vi "Automatic Frequency Linearization.vi"() -> ()   [LabVIEW 2014]
panel:
  out "1) Falling Max-Min error Graph":cluster{dbl[], dbl[]}(graph)
  out "2) Rising Max-Min error Graph":cluster{dbl[], dbl[]}(graph)
  out "2) Rising Max-Min error %":dbl
  out "1) Falling Max-Min error %":dbl
  in  "Active PolyFit of Mean Freq":bool
  out "Triangular skewtri generated from min factor":dbl[](graph)
  in  "Sample /Modulation Frequency":enum32{"40MHz/32KHz", "30MHz/24Khz"}(radio)=enum."30MHz/24Khz"
  in  "Scaling factor":dbl=1.0
  out "Rising Min Factor":dbl
  out "Falling Min Factor":dbl
  out "Rising Min DevStd%":dbl
  out "Falling Min DevStd%":dbl
  out "Fine?":bool
  out "Ok?":bool
  in  "#MeanMeasuraments":i32=50
  in  "StopValue":dbl=0.2
  in  "stop":bool
  out "Mean  FREQUENCY Curve Falling":dbl[](graph)
  out "Mean FREQUENCY Curve Rising":dbl[](graph)
  out "Current Skew Tri":dbl[](graph)
  out "Current Mul factor":dbl
  out "Current iteration (Countdown)":dbl
  out "Rising<= 1%":bool
  out "Falling<= 1%":bool
  in  "DeltaFactor":dbl=0.01
  in  "Initial Factor Mul":dbl=0.35
  out "2) Rising StdDev % Graph":cluster{dbl[], dbl[]}(graph)
  out "1) Falling StdDev % Graph":cluster{dbl[], dbl[]}(graph)
  out "2) Rising Std Dev %":dbl
  out "1) Falling Std Dev %":dbl
  out "2) Rising Signal (Last)":dbl[](graph)
  out "1) Falling Signal (Last)":dbl[](graph)
  in  "#LinMesuraments":i32=20
  # "OFFLINE SETUP"
  # "CURRENT ITERATION"
  # "Fattore moltiplicativo"
  # "Numero di misure su cui calcolare la curva delle frequenze medie con triangolo dritto"
  # "Numero di misurazioni\n su cui mediare durante la\nlinearizzazione"
  # "Optimal Factor Rising: 0.33    with Falling curve: 0.294"
  # "Optimal Factor Falling: 0.22/0.23"
  # "Fattore moltiplicativo\nIniziale"
  # "Passo del fattore\nmoltiplicativo"
  # "Fattore moltiplicativo\nFinale"
  # "%"
  # "%"
  # "FINAL RESULTS"
  # "Andamento della deviazione standard percentuale in funzione del fattore moltiplicativo"
  # "%"
  # "%"
  # "min 0,27"
  # "min 0,16"
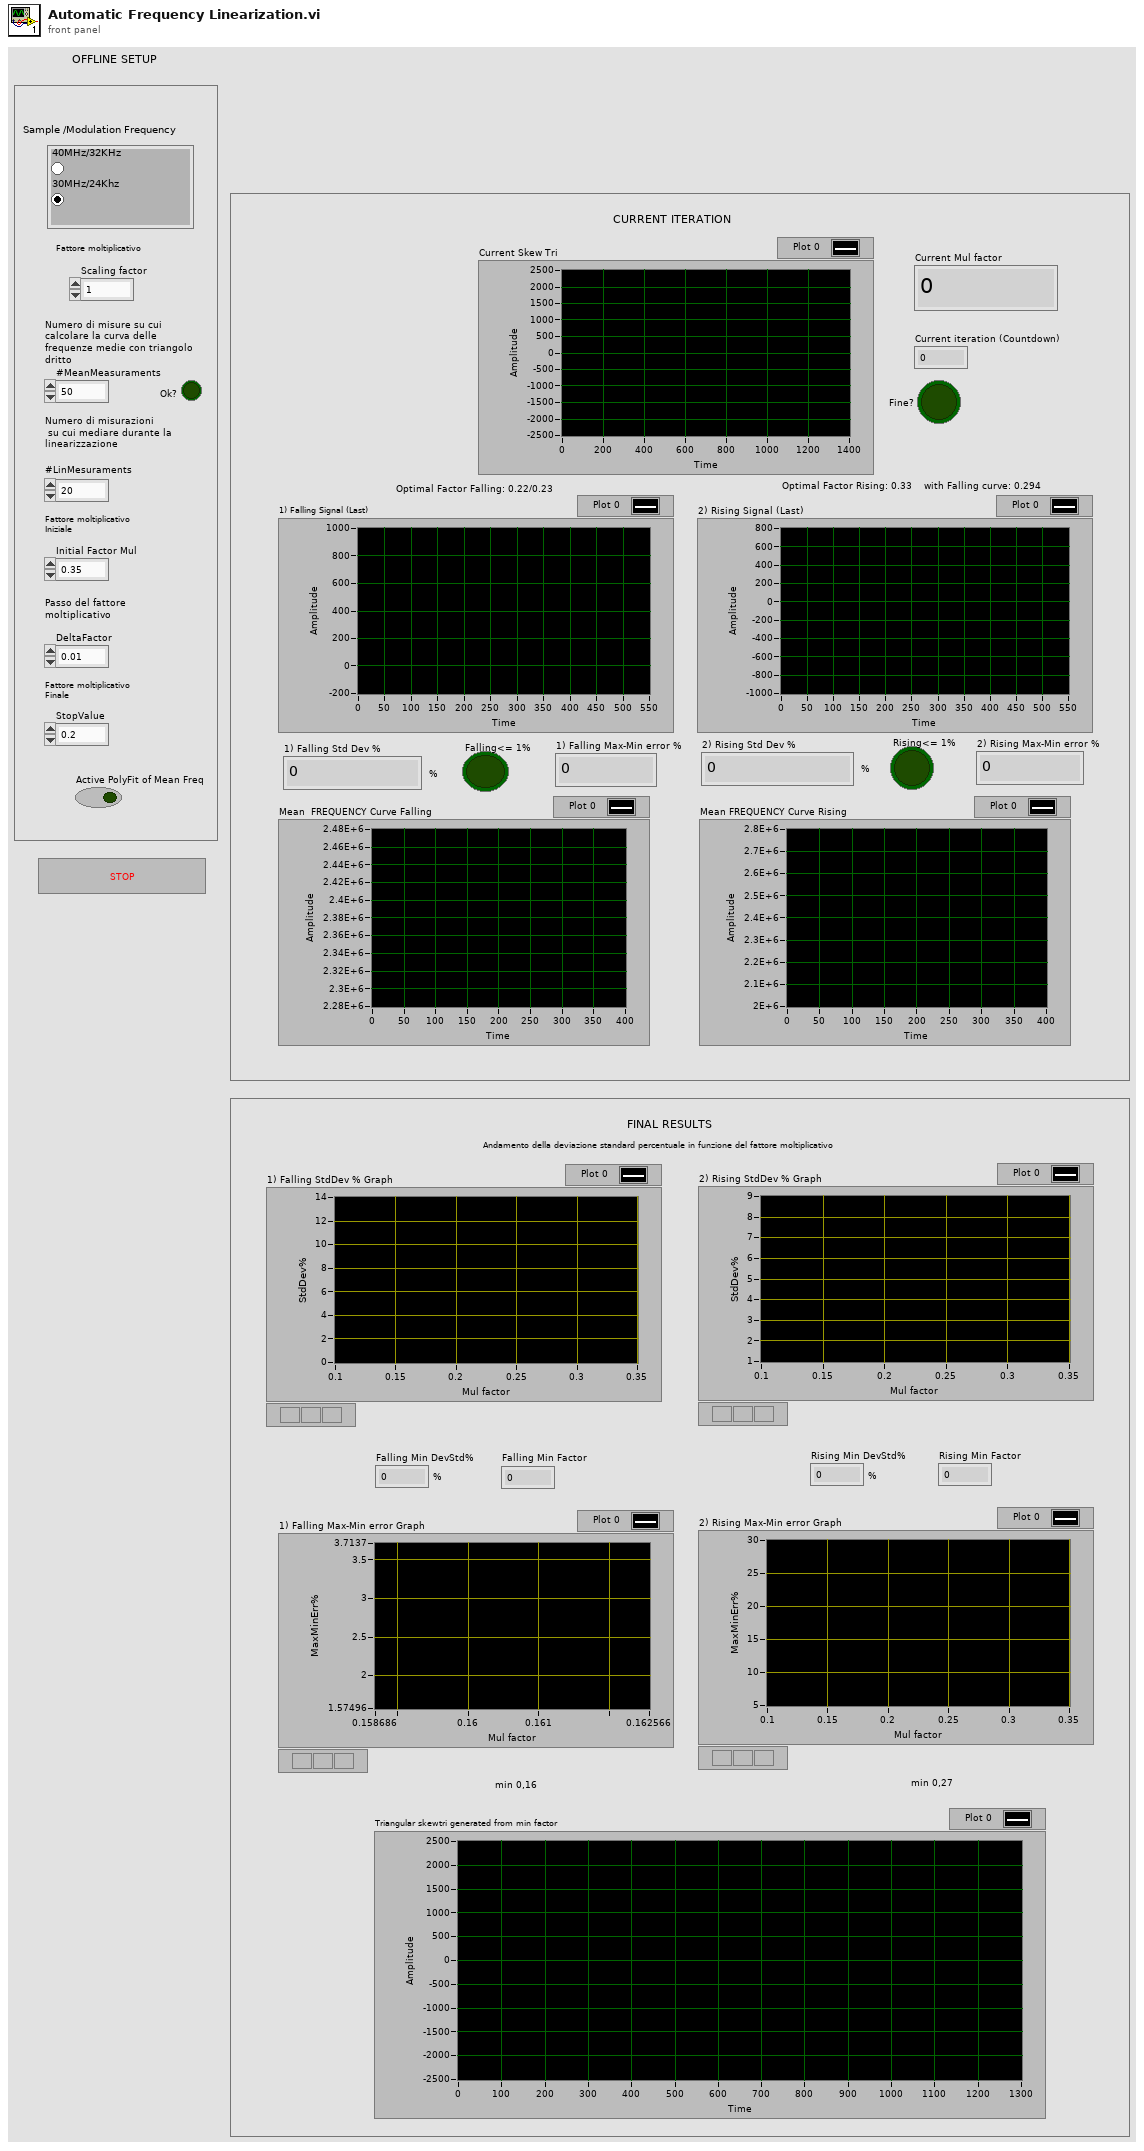
[diagram p1: front panel]
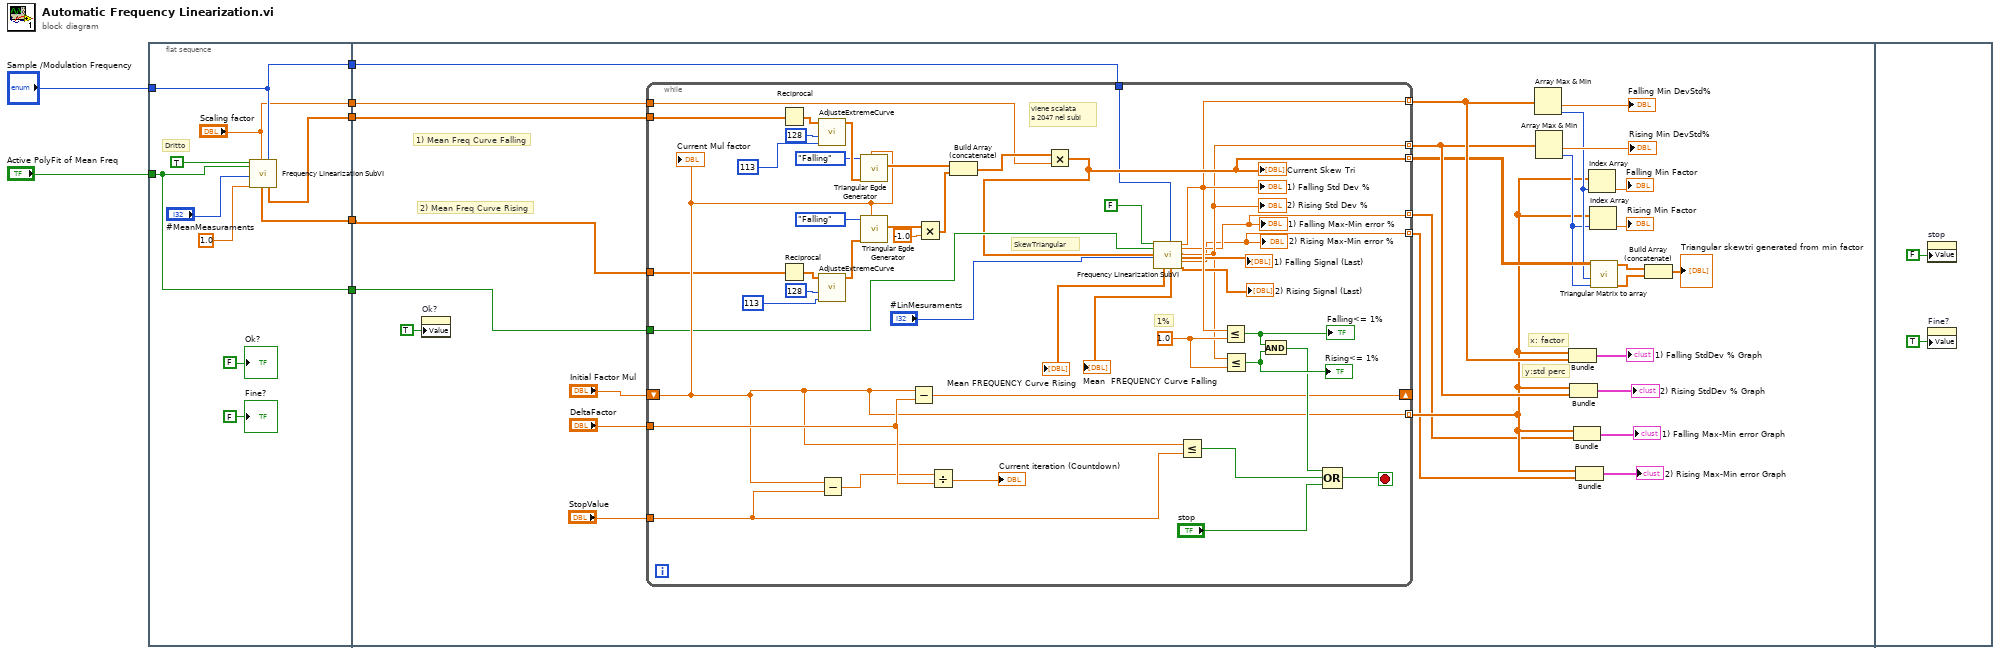
[diagram p0: block diagram]
diagram:
  n1 = flat-sequence {
    tunnel: [w14] -> w7
    tunnel: [w13] -> w6
    tunnel: ["Scaling factor"] -> w5
    tunnel: "Sample /Modulation Frequency" -> [w15]
    tunnel: [w15] -> w3
    tunnel: "Active PolyFit of Mean Freq" -> [w8]
    tunnel: [w8] -> w1
    tunnel: w7 -> [w32]
    tunnel: w6 -> [w33]
    tunnel: w5 -> [w31]
    tunnel: w3 -> [w30]
    tunnel: w1 -> [w23]
    frame #0 {
      # "Dritto"
      n2 = call "Frequency Linearization SubVI.vi"("Triangolo dritto"=TRUE, "Active PolyFit"=w8, "#Medie"="#MeanMeasuraments", "Scale factor"=1.0, "Scaling factor"="Scaling factor", "Sample /Modulation Frequency"=w15) -> ("Last Mean Freq Curve Rising"=w13:dbl[], "Last Mean Freq Curve Falling"=w14:dbl[])  [unwired: 6 in, 6 out]
      "Ok?" <- FALSE ("Ok?")
      "Fine?" <- FALSE ("Ok?")
    }
    frame #1 {
      # "2) Mean Freq Curve Rising"
      # "1) Mean Freq Curve Falling"
      # "y:std perc"
      # "x: factor"
      n3 = property on="Ok?" class="Bool (strict)"("Value"=TRUE ("Ok?")) -> ()  [unwired: 2 in, 2 out]
      n4 = while {
        tunnel: [w51] -> w39 mode=indexing
        tunnel: [w48] -> w36 mode=indexing
        shift-right: [w68] -> _
        shift-left: "Initial Factor Mul" -> [w65]
        tunnel: "DeltaFactor" -> [w66]
        tunnel: w32 -> [w60]
        tunnel: w33 -> [w59]
        tunnel: [w65] -> w22 mode=indexing
        tunnel: "StopValue" -> [w64]
        tunnel: w31 -> [w61]
        tunnel: w30 -> [w54]
        tunnel: [w56] -> w29 mode=indexing
        tunnel: w23 -> [w57]
        tunnel: [w47] -> w21 mode=indexing
        tunnel: [w46] -> w20 mode=indexing
        stop <- w71 stop-if-true
        w88 = 1.0 ("y")
        # "viene scalata \na 2047 nel subi"
        # "SkewTriangular"
        # "1%"
        n5 = Reciprocal(x=w60) -> (1/x=w75:dbl[])
        n6 = Reciprocal(x=w59) -> (1/x=w86:dbl[])
        n7 = call "AdjusteExtremeCurve.vi"("Init Bins Discarded"=u32 113, "FFT Size Window"=128, "Freq sample"=w75) -> ("Extended Freq Sample"=w79:dbl[])  [unwired: 8 in]
        n8 = call "AdjusteExtremeCurve.vi"("Init Bins Discarded"=u32 113, "FFT Size Window"=128, "Freq sample"=w86) -> ("Extended Freq Sample"=w80:dbl[])  [unwired: 8 in]
        n9 = Subtract(x=w65, y=w64) -> (x-y=w63:dbl)
        n10 = call "Triangular Egde Generator.vi"("fattore"=w65, "Sample values"=w79, "Triangular edge"=enum16{"Rising", "Falling"}."Falling") -> ("Skew Triangular"=w78:dbl[])  [unwired: 8 in]
        n11 = call "Triangular Egde Generator.vi"("fattore"=w65, "Sample values"=w80, "Triangular edge"=enum16{"Rising", "Falling"}."Falling") -> ("Skew Triangular"=w82:dbl[])  [unwired: 8 in]
        n12 = Subtract(x=w65, y=w66) -> (x-y=w68:dbl)
        n13 = Multiply(x=w82, y=-1.0) -> (x*y=w83:dbl[])
        n14 = Divide(x=w63, y=w66) -> (x/y=→"Current iteration (Countdown)":dbl)
        n15 = Build Array (concatenate)(w78, w83) -> (w62:dbl[])
        n16 = Multiply(x=w62, y=w61) -> (x*y=w56:dbl[])
        "Current Skew Tri" <- w56
        n17 = call "Frequency Linearization SubVI.vi"("Triangolo dritto"=FALSE, "Active PolyFit"=w57, "Sketri Input"=w56, "#Medie"="#LinMesuraments", "Sample /Modulation Frequency"=w54) -> ("Last Mean Freq Curve Rising"=→"Mean FREQUENCY Curve Rising":dbl[], "Last Mean Freq Curve Falling"=→"Mean  FREQUENCY Curve Falling":dbl[], "Falling Std Dev %"=w51:dbl, "Falling Max-Min error (% over Mean)"=w47:dbl, "Rising Std Dev %"=w48:dbl, "First Signal (Last)"=→"1) Falling Signal (Last)":dbl[], "Rising Max-Min error (% over Mean)"=w46:dbl, "Second Signal (Last)"=→"2) Rising Signal (Last)":dbl[])  [unwired: 7 in]
        "1) Falling Std Dev %" <- w51
        "2) Rising Std Dev %" <- w48
        "1) Falling Max-Min error %" <- w47
        "2) Rising Max-Min error %" <- w46
        n18 = Less Or Equal?(x=w65, y=w64) -> (x <= y?=w67:bool)
        n19 = Less Or Equal?(x=w51, y=w88) -> (x <= y?=w89:bool)
        "Falling<= 1%" <- w89
        n20 = Less Or Equal?(x=w48, y=w88) -> (x <= y?=w87:bool)
        "Rising<= 1%" <- w87
        n21 = And(x=w89, y=w87) -> (x .and. y?=w70:bool)
        n22 = Compound Arithmetic op=OR(w70, w67, "stop") -> (w71:bool)
        "Current Mul factor" <- w65
      }
      n23 = Array Max & Min(array=w39) -> (min value=→"Falling Min DevStd%":dbl, min index (indices)=w28:i32)  [unwired: 2 out]
      n24 = Array Max & Min(array=w36) -> (min value=→"Rising Min DevStd%":dbl, min index (indices)=w27:i32)  [unwired: 2 out]
      n25 = Bundle(w22, w39) -> (→"1) Falling StdDev % Graph":cluster{dbl[], dbl[]})  [unwired: 1 in]
      n26 = Bundle(w22, w36) -> (→"2) Rising StdDev % Graph":cluster{dbl[], dbl[]})  [unwired: 1 in]
      n27 = Bundle(w22, w21) -> (→"1) Falling Max-Min error Graph":cluster{dbl[], dbl[]})  [unwired: 1 in]
      n28 = Bundle(w22, w20) -> (→"2) Rising Max-Min error Graph":cluster{dbl[], dbl[]})  [unwired: 1 in]
      n29 = Index Array(array=w22, index=w28) -> (element=→"Falling Min Factor":dbl)
      n30 = Index Array(array=w22, index=w27) -> (element=→"Rising Min Factor":dbl)
      n31 = call "Triangular Matrix to array.vi"("index second subarray"=w27, "index first subarray"=w28, "Array"=w29) -> ("Array second"=w25:dbl[], "Array first"=w26:dbl[])  [unwired: 7 in]
      n32 = Build Array (concatenate)(w26, w25) -> (→"Triangular skewtri generated from min factor":dbl[])
    }
    frame #2 {
      n33 = property on="stop" class="Bool (strict)"("Value"=FALSE ("stop")) -> ()  [unwired: 2 in, 2 out]
      n34 = property on="Fine?" class="Bool (strict)"("Value"=TRUE ("Fine?")) -> ()  [unwired: 2 in, 2 out]
    }
  }
